vi "Convert Unicode to ASCII.vi"(4 "Unicode String In":string) -> (0 "ASCII":bool, 1 "ASCII String Out":string)   [LabVIEW 2012]
doc: "Convert a Unicode string to ASCII.\n\nChristopher G. Relf\nCertified LabVIEW Architect\nchristopher_relf@yahoo.com\nCopyright (c) 2004 - All Rights Reserved\n\nLicense:\nThis code is owned by Christopher G. Relf and is licensed under the Creative Commons License. See http://creativecommons.org for full license terms.\n\nThis VI is LAVA Certified. For more information, visit http://forums.lavag.org."
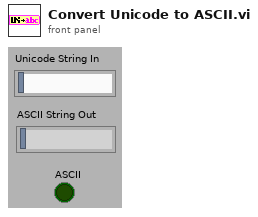
[diagram p1: front panel]
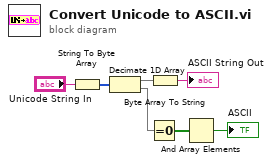
[diagram p0: block diagram]
diagram:
  n1 = String To Byte Array(string="Unicode String In") -> (unsigned byte array=w5:u8[])
  n2 = Decimate 1D Array(w5) -> (w4:u8[], w3:u8[])
  n3 = Equal To 0?(x=w3) -> (x = 0?=w2:bool[])
  n4 = Byte Array To String(unsigned byte array=w4) -> (string=→"ASCII String Out":string)
  n5 = And Array Elements(Boolean array=w2) -> (logical AND=→"ASCII":bool)
